vi "ResetEC.vi"   [LabVIEW 2015]
uses:
  ESLSCDLL.dll
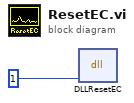
[diagram p0: block diagram]
diagram:
  n1 = dll-call lib="C:/ENTW/PCIE/lv64/board.vis/ESLSCDLL.dll" fn="DLLResetEC" ("lwlscdll.dll:DLLSetTemp")("drv"=u32 1) -> ()  [unwired: 5 in, 2 out]
